vi "R2T_Iter.vi"(2 "T-Ziel":dbl=2.560777925500073 format="%.5f") -> (1 "R":dbl=22.359058380126953 format="%.2f")   [LabVIEW 2010]
uses:
  Instrument_Setup.vi
panel:
  out "Durchläufe":dbl=112500.0 format="%.2f"
  out "delta":dbl=0.455774097521615 format="%.6f"
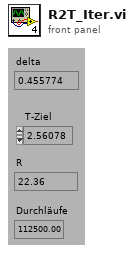
[diagram p1: front panel]
types:
  T1 = cluster{"R start":dbl, "R warm":dbl, "R kalt":dbl}[]
  T2 = cluster{"R start":dbl, "R warm":dbl, "R kalt":dbl}
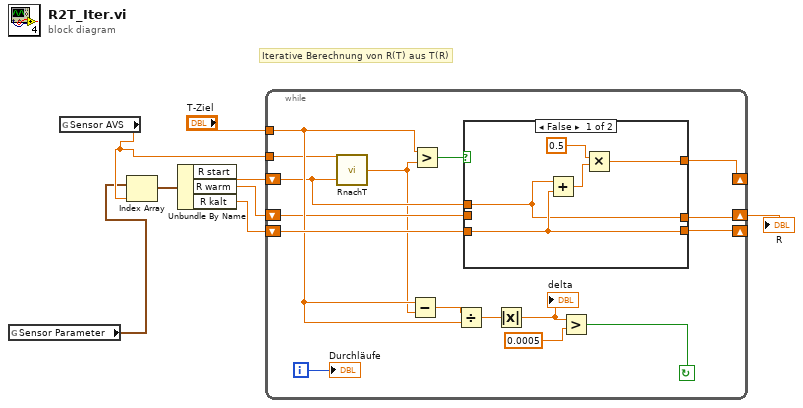
[diagram p0: block diagram]
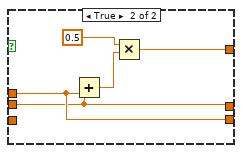
[diagram p2: hidden frame]
diagram:
  # "Iterative Berechnung von R(T) aus T(R)"
  n1 = global read "Instrument_Setup.vi" "Sensor Parameter"() -> (w1:T1)
  n2 = global read "Instrument_Setup.vi" "Sensor AVS"() -> (w2:dbl)
  n3 = Index Array(array=w1, index=w2) -> (element=w3:T2)
  n4 = Unbundle By Name(w3) -> ("R start"=w4:dbl, "R warm"=w5:dbl, "R kalt"=w6:dbl)
  n5 = while {
    tunnel: w2 -> [w10]
    shift-left: w4 -> [w11]
    shift-right: [w14] -> _
    shift-left: w6 -> [w22]
    shift-right: [w21] -> _
    tunnel: "T-Ziel" -> [w15]
    shift-left: w5 -> [w13]
    shift-right: [w12] -> w7
    i -> [w24]
    stop <- w16 continue-if-true
    n6 = call "RnachT.vi"("R"=w11, "Sensor Cal #"=w10) -> ("T (K)"=w9:dbl)
    n7 = Subtract(x=w15, y=w9) -> (x-y=w20:dbl)
    n8 = Greater?(x=w15, y=w9) -> (0:w23:bool)
    n9 = Divide(x=w20, y=w15) -> (x/y=w19:dbl)
    n10 = case shown="False" w23 {
      tunnel: w11 -> [w25 w31]
      tunnel: w22 -> [w26 _]
      tunnel: [w26 w31] -> w21
      tunnel: [w27 w34] -> w14
      tunnel: w13 -> [_ w30]
      tunnel: [w25 w30] -> w12
      frame False {
        n11 = Add(x=w25, y=w26) -> (x+y=w29:dbl)
        n12 = Multiply(x=0.5, y=w29) -> (x*y=w27:dbl)
      }
      frame True {
        n13 = Add(x=w31, y=w30) -> (x+y=w32:dbl)
        n14 = Multiply(x=0.5, y=w32) -> (x*y=w34:dbl)
      }
    }
    n15 = Absolute Value(x=w19) -> (abs(x)=w17:dbl)
    "delta" <- w17
    n16 = Greater?(x=w17, y=0.0005) -> (0:w16:bool)
    "Durchläufe" <- w24
  }
  "R" <- w7
